vi "Init.vi"(8 "error in (no error)":errorcluster, 11 "Data in":refnum<class "Double Float Array 1D.lvclass">) -> (0 "error out":errorcluster, 3 "Data out":refnum<class "Double Float Array 1D.lvclass">)   [LabVIEW 2021, in "Variable.lvlib" / "Double Float Array 1D.lvclass"]
uses:
  Double Float Array 1D.lvclass
  Double Float Array 1D.lvclass/Double Float Array 1D.ctl
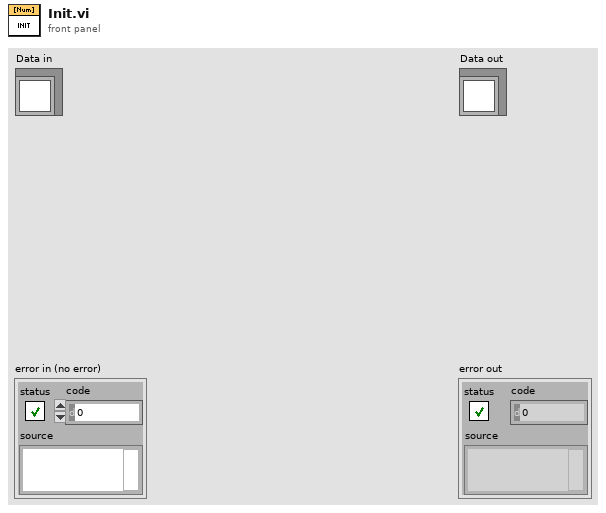
[diagram p1: front panel]
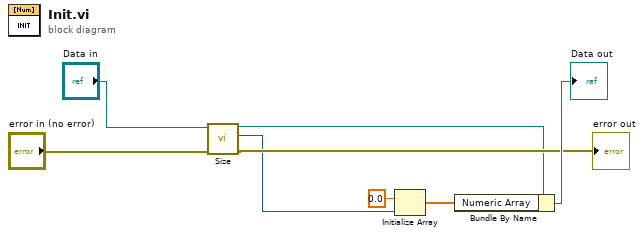
[diagram p0: block diagram]
diagram:
  n1 = call-dynamic "Size.vi"("error in (no error)"="error in (no error)", "Vector Parent in"="Data in") -> ("error out"=→"error out":errorcluster, "size"=w1:i32, "Vector Parent out"=w2:refnum<class "Double Float Array 1D.lvclass">)  [unwired: 7 in]
  n2 = Initialize Array(0.0 ("element"), w1) -> (w6:dbl[])
  n3 = Bundle By Name(cluster=w2, "Numeric Array"=w6) -> (→"Data out":refnum<class "Double Float Array 1D.lvclass">)
